vi "destroy.vi"(8 "error in (no error)":errorcluster, 11 "ImageCollection in":refnum<class "ImageCollection.lvclass">) -> (0 "error out":errorcluster, 3 "ImageCollection out":refnum<class "ImageCollection.lvclass">)   [LabVIEW 2010, in "ImageCollection.lvclass"]
uses:
  ImageCollection.lvclass
  Image/Image/Image.lvclass
  ImageCollection.lvclass/ImageCollection.ctl
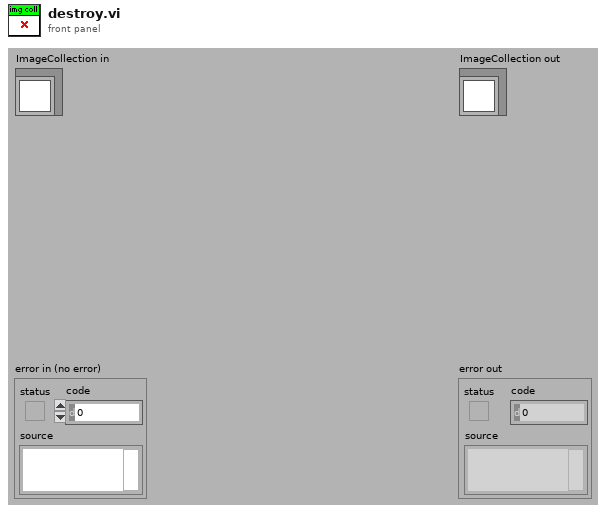
[diagram p1: front panel]
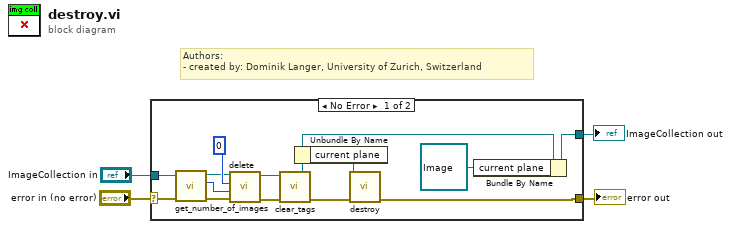
[diagram p0: block diagram]
diagram:
  # "Authors: \n- created by: Dominik Langer, University of Zurich, Switzerland"
  n1 = case shown="No Error" "error in (no error)" {
    selector: "error in (no error)" -> [w17 w20]
    tunnel: [w9 w20] -> w3
    tunnel: [w6 w19] -> w1
    tunnel: "ImageCollection in" -> [w14 w19]
    frame No Error {
      n2 = call-dynamic "get_number_of_images.vi"("error in (no error)"=w17, "ImageCollection in"=w14) -> ("error out"=w16:errorcluster, "size"=w15:i32, "ImageCollection out"=w13:refnum<class "ImageCollection.lvclass">)  [unwired: 7 out]
      n3 = call-dynamic "delete.vi"("error in (no error)"=w16, "range"=w15, "start index"=0, "ImageCollection in"=w13) -> ("error out"=w12:errorcluster, "ImageCollection out"=w11:refnum<class "ImageCollection.lvclass">)  [unwired: 6 out]
      n4 = call "clear_tags.vi"("error in (no error)"=w12, "ImageCollection in"=w11) -> ("error out"=w10:errorcluster, "ImageCollection out"=w7:refnum<class "ImageCollection.lvclass">)  [unwired: 8 in]
      n5 = Unbundle By Name(w7) -> ("current plane"=w8:refnum<class "Image.lvclass">)
      n6 = call-dynamic "destroy.vi"("error in (no error)"=w10, "Image in"=w8) -> ("error out"=w9:errorcluster)  [unwired: 8 in, 1 out]
      n7 = Bundle By Name(cluster=w7, "current plane"=refnum<class "Image.lvclass"> refnum) -> (w6:refnum<class "ImageCollection.lvclass">)
    }
    frame Error {
    }
  }
  "error out" <- w3
  "ImageCollection out" <- w1
